vi "TestExec.Append Fault Code Prefix.vi"(7 "Positive(F)\\Negative(T)":bool, 9 "FaultCode":i32, 10 "FaultCode Prefix":i32) -> (1 "New Fault Code":i32)   [LabVIEW 2019]
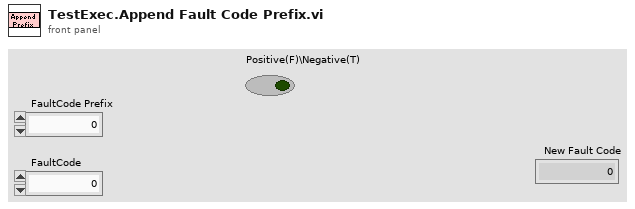
[diagram p1: front panel]
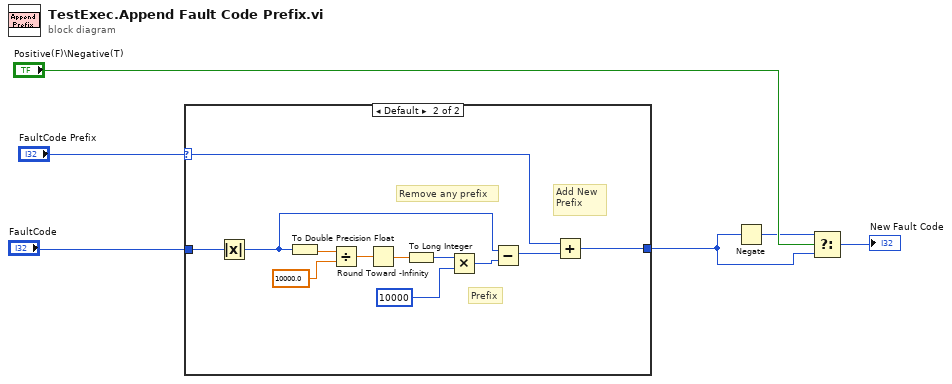
[diagram p0: block diagram]
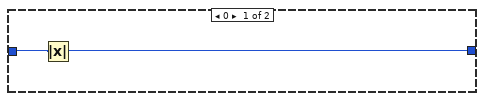
[diagram p2: hidden frame]
diagram:
  n1 = case shown="Default" "FaultCode Prefix" {
    selector: "FaultCode Prefix" -> [_ w12]
    tunnel: "FaultCode" -> [w8 w11]
    tunnel: [w7 w9] -> w2
    frame 0 {
      n2 = Absolute Value(x=w8) -> (abs(x)=w7:i32)
    }
    frame Default {
      # "Add New\nPrefix"
      # "Remove any prefix"
      # "Prefix"
      n3 = Absolute Value(x=w11) -> (abs(x)=w10:i32)
      n4 = To Double Precision Float(number=w10) -> (double precision float=w20:dbl)
      n5 = Divide(x=w20, y=10000.0) -> (x/y=w18:dbl)
      n6 = Round Toward -Infinity(1:w18) -> (0:w17:dbl)
      n7 = To Long Integer(number=w17) -> (32bit integer=w16:i32)
      n8 = Multiply(x=w16, y=10000) -> (x*y=w14:i32)
      n9 = Subtract(x=w10, y=w14) -> (x-y=w13:i32)
      n10 = Add(x=w12, y=w13) -> (x+y=w9:i32)
    }
  }
  n11 = Negate(x=w2) -> (-x=w4:i32)
  n12 = Select(t=w4, s="Positive(F)\\Negative(T)", f=w2) -> (s? t:f=→"New Fault Code":i32)
